vi "main.vi"() -> ()   [LabVIEW 2021]
uses:
  Controls/App Data Cluster.ctl
  Controls/UI Reference Cluster.ctl
  Controls/Database Variables Cluster.ctl
  <vilib>/drjdpowell/SQLite Library/SQL Connection/Connection.lvclass
  <vilib>/drjdpowell/SQLite Library/SQL Connection/Open (string).vi
  <extravilib>/ChannelInstances/Event Messenger-c(str,var)/Instantiate.vi
  <extravilib>/ChannelInstances/Event Messenger-c(str,var)/))Channel.vi
  <vilib>/drjdpowell/SQLite Library/SQL Connection/Execute SQL (1D DBL results).vi
  <vilib>/drjdpowell/SQLite Library/SQL Connection/Execute SQL (No results).vi
  <vilib>/Instr/_visa.llb/VISA Configure Serial Port (Instr).vi
  <extravilib>/ChannelInstances/Event Messenger-c(str,var).lvlib
  <vilib>/drjdpowell/SQLite Library/SQLite.lvlib
  <vilib>/JDP Science/JDP Science Common Utilities/JDP Utility.lvlib
panel:
  out "EndTime":string
  out "Result Set":dbl[](array[numeric])
  out "MDBUnit Test Result":cluster{"Message":string, "Passed?":bool}
  in  "Python script path":path=path "C:/Isaac/Projects/Mechanical Engineering Projects/LabVIEW Databases Project/LabVIEW-Databases/Python/mdb_helper.py"
  in  "Python install path":path=path "C:/Users/RIG/AppData/Local/Programs/Python/Python39-32/python.exe"
  out "SQLite Write Test Result":cluster{"Message":string, "Passed?":bool}
  in  "SQLite DB Path":string="C:\\Isaac\\Projects\\Mechanical Engineering Projects\\LabVIEW Databases Project\\SensorsDB.db"
  out "Serial Read Unit test results":cluster{"message":string, "Passed?":bool}[](array[cluster])
  out "App Data - Database Loop":T1
  out "error out":errorcluster
  in  "Save to MongoDB?":bool
  in  "Confirm details":bool
  in  "Save to SQLite?":bool
  in  "Start":bool
  in  "Stop":bool
  in  "Config run":bool
  in  "Select VISA resource name":refnum<visa-resource-name>
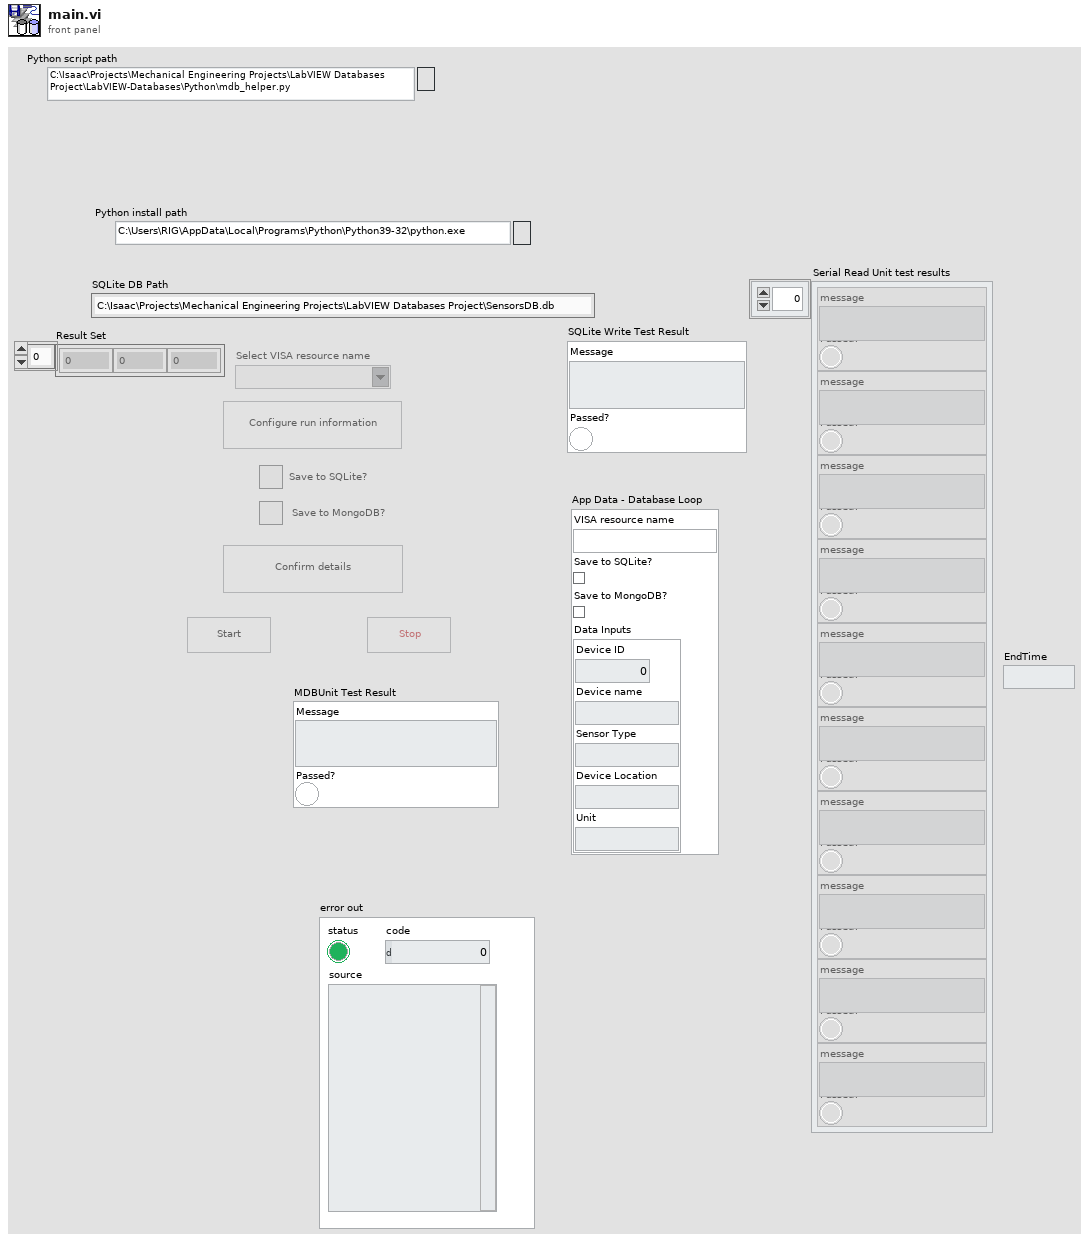
[diagram p1: front panel]
types:
  T1 = typedef "App Data Cluster.ctl" = cluster{"VISA resource name":refnum<visa-resource-name>, "Save to SQLite?":bool, "Save to MongoDB?":bool, "Data Inputs":cluster{"Device ID":dbl, "Device name":string, "Sensor Type":string, "Device Location":string, "Unit":string}}
  T2 = typedef "Database Variables Cluster.ctl" = cluster{"SQLite Connection":refnum<class "Connection.lvclass">, "Python Session":refnum<k35>, "Duplicate SQLite?":bool, "Duplicate MongoDB?":bool, "Start Time":string}
  T3 = typedef "UI Reference Cluster.ctl" = cluster{"Select VISA resource name":refnum<vi>, "Config run":refnum<vi>, "Save to SQLite":refnum<vi>, "Save to MongoDB":refnum<vi>, "Confirm details":refnum<vi>, "Start":refnum<vi>, "Stop":refnum<vi>}
  T4 = typedef "Event Messenger-c(str,var).lvlib/))Channel.ctl" = refnum<queue>
  T5 = cluster{"Device ID":dbl, "Device name":string, "Sensor Type":string, "Device Location":string, "Unit":string}
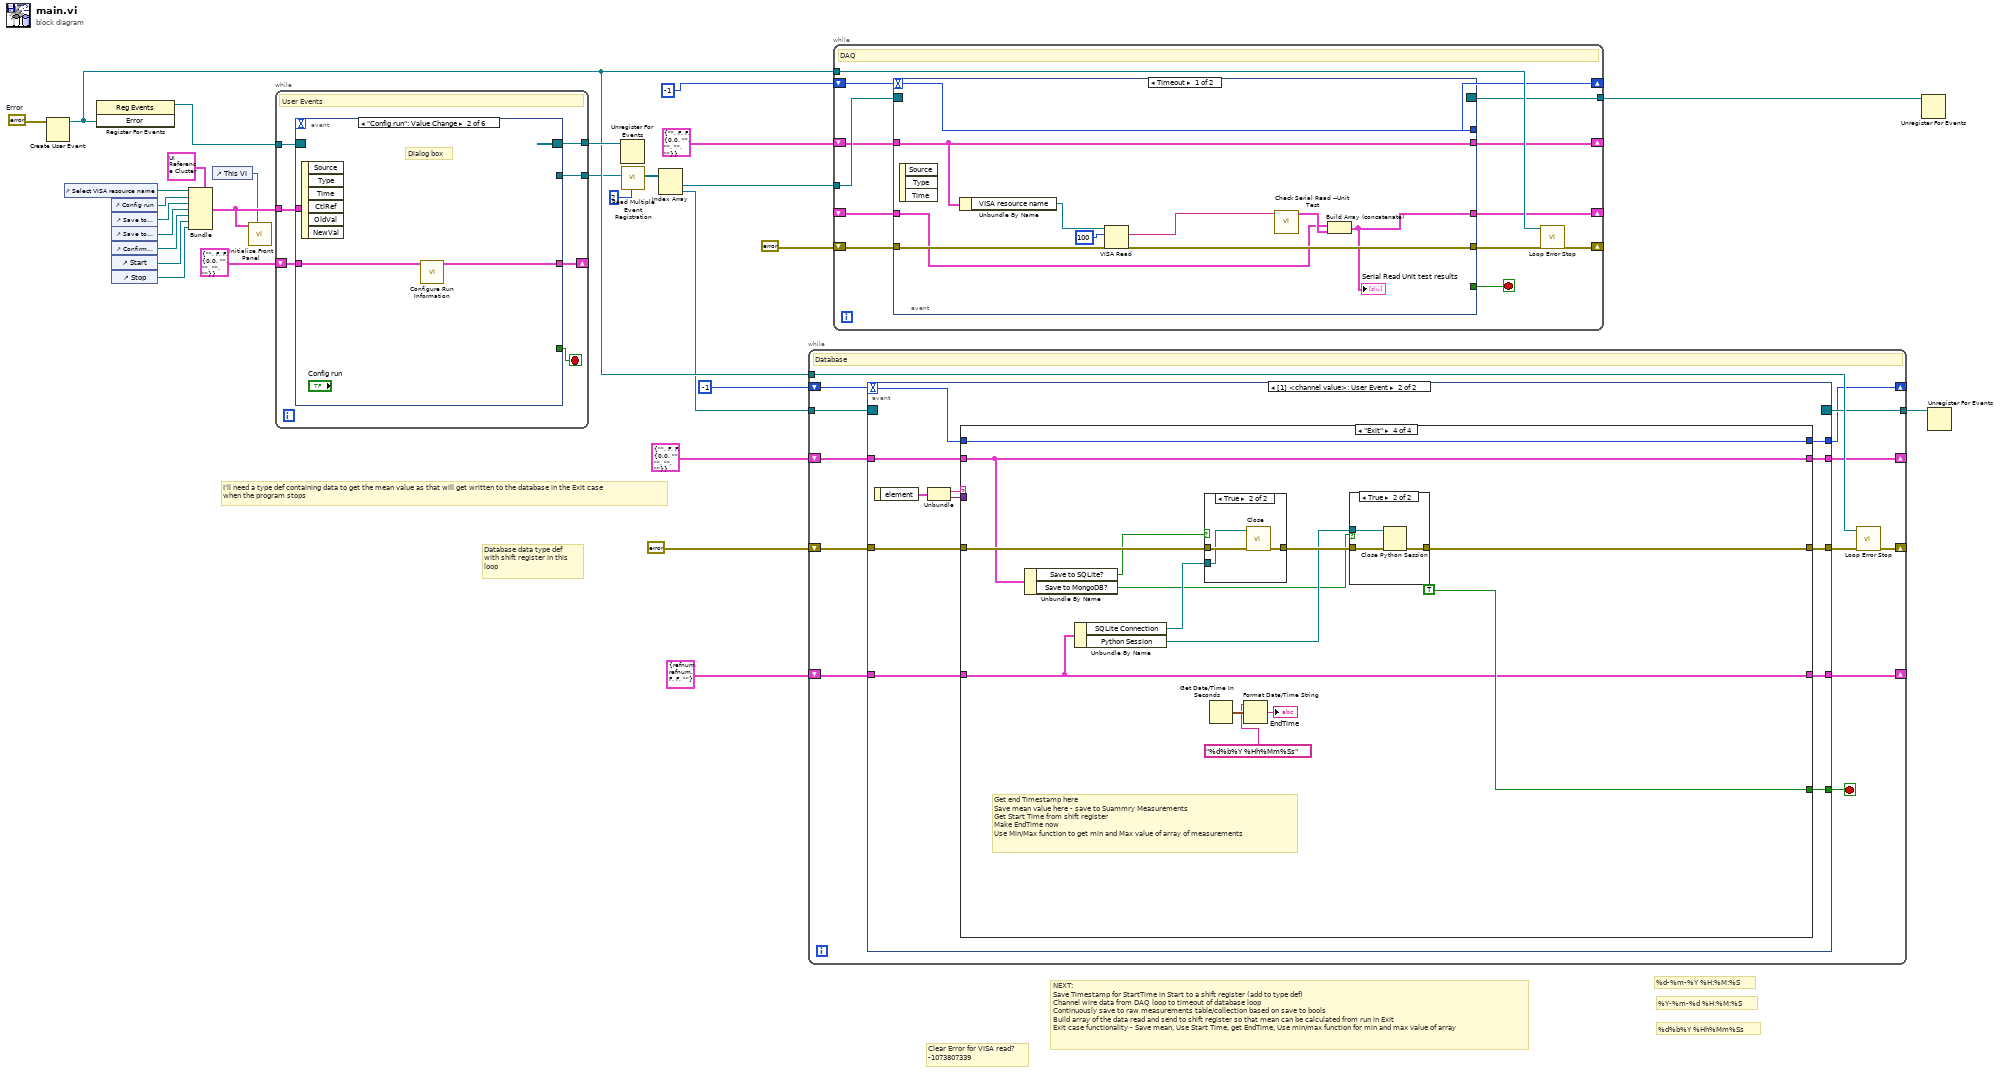
[diagram p0: block diagram]
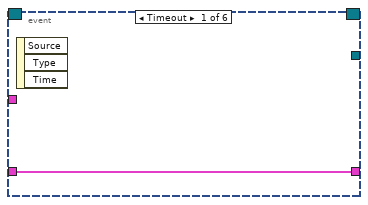
[diagram p2: hidden frame]
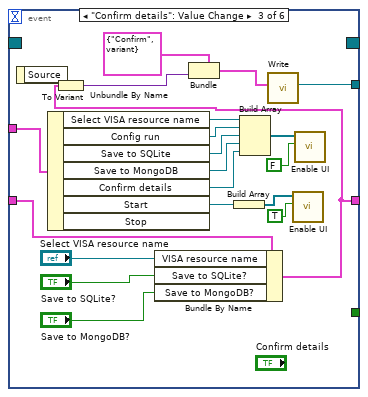
[diagram p3: hidden frame]
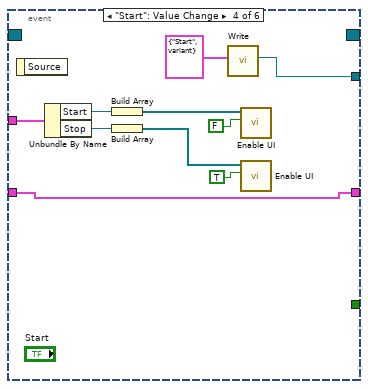
[diagram p4: hidden frame]
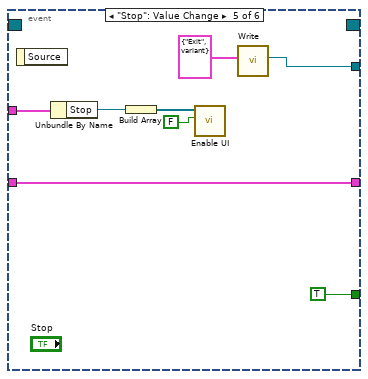
[diagram p5: hidden frame]
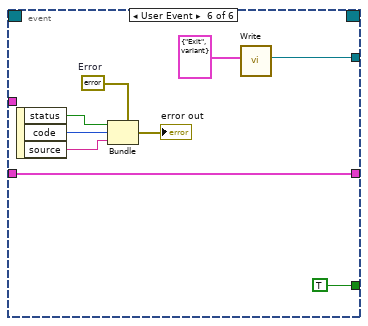
[diagram p6: hidden frame]
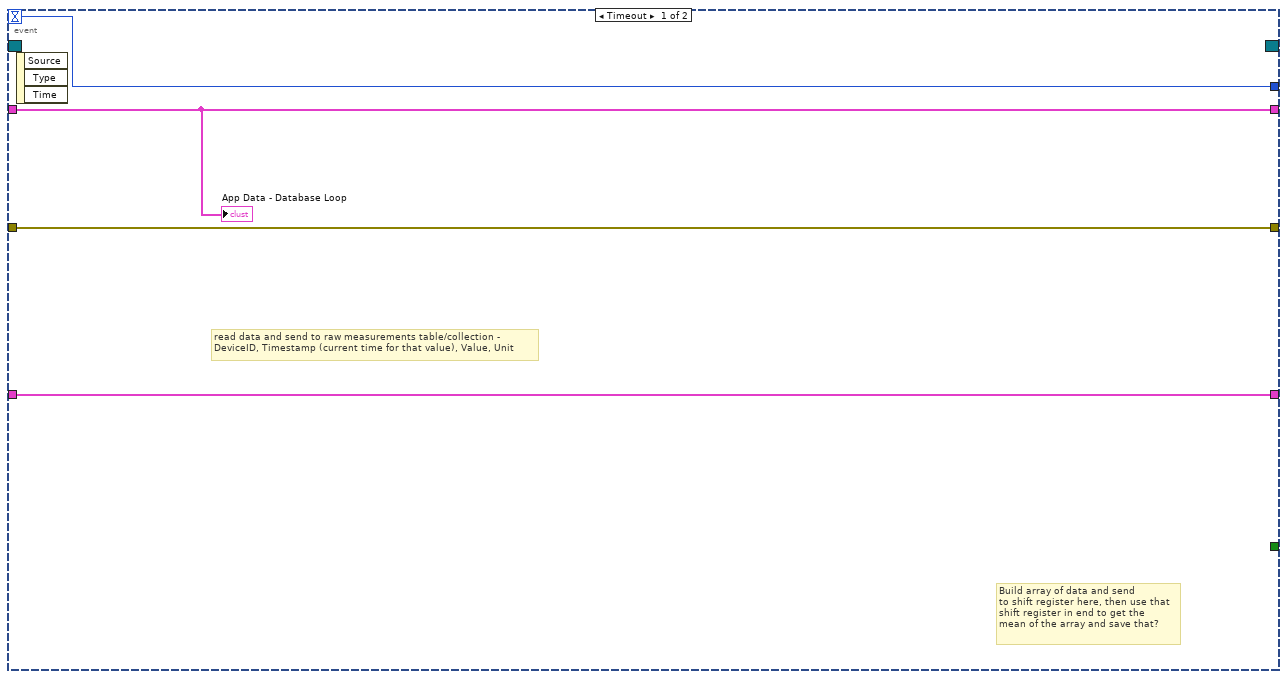
[diagram p7: hidden frame]
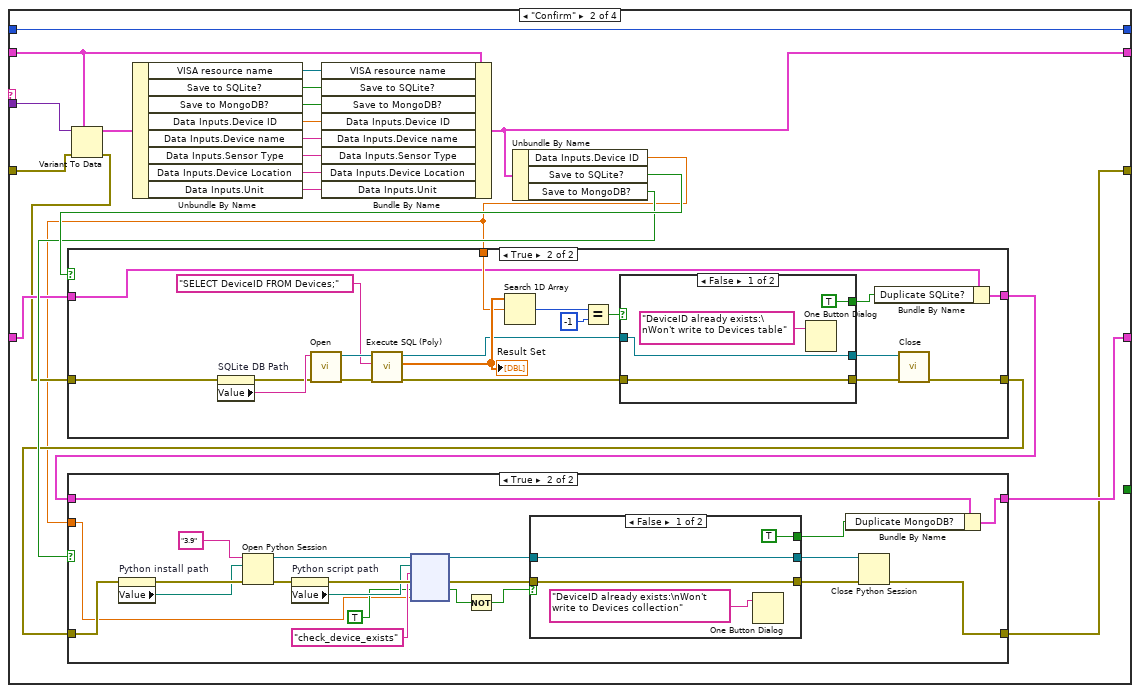
[diagram p9: hidden frame]
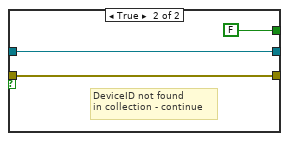
[diagram p11: hidden frame]
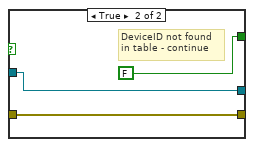
[diagram p13: hidden frame]
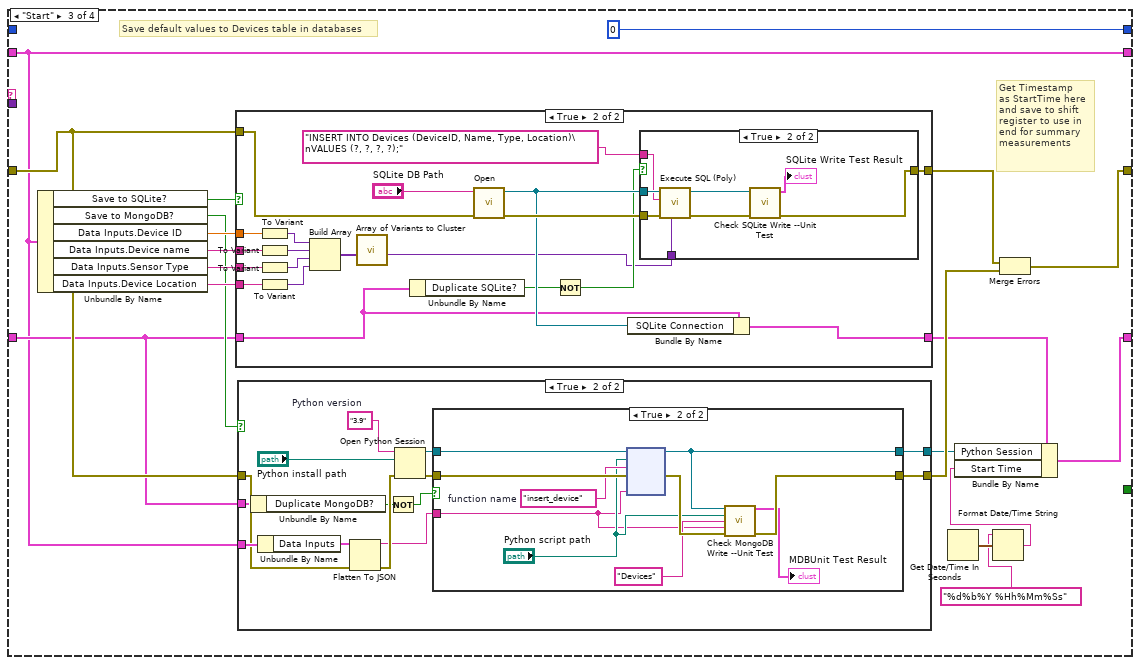
[diagram p14: hidden frame]
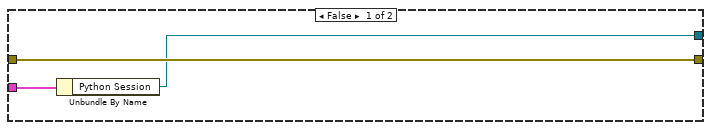
[diagram p15: hidden frame]
diagram:
  w22 = errorcluster {"status"=FALSE, "code"=0, "source"=""}  # Error
  # "%d-%m-%Y %H:%M:%S"
  # "%d%b%Y %Hh%Mm%Ss"
  # "%Y-%m-%d %H:%M:%S"
  # "Clear Error for VISA read?\n-1073807339"
  # "NEXT:\nSave Timestamp for StartTime in Start to a shift register (add to type def)\nChannel wire data from DAQ loop to timeout of database loop\nContinuously save to raw measurements table/collection based on save to bools\nBuild array of the data read and send to shift register so that mean can be calculated from run in Exit\nExit case functionality - Save mean, Use Start Time, get EndTime, Use min/max function for min and max value of array"
  # "Database data type def\nwith shift register in this \nloop"
  # "I'll need a type def containing data to get the mean value as that will get written to the database in the Exit case\nwhen the program stops"
  n1 = Create User Event(user event datatype=w22) -> (user event=w19:refnum<user-event>)  [unwired: 1 in, 1 out]
  n2 = control-ref of="Select VISA resource name"() -> (w29:refnum<vi>)
  n3 = register-events(w19) -> (reference out=w21:refnum<event-registration>)  [unwired: 2 in, 1 out]
  n4 = control-ref of="Config run"() -> (w28:refnum<vi>)
  n5 = control-ref of="Save to SQLite?"() -> (w27:refnum<vi>)
  n6 = control-ref of="Save to MongoDB?"() -> (w26:refnum<vi>)
  n7 = control-ref of="Confirm details"() -> (w25:refnum<vi>)
  n8 = control-ref of="Start"() -> (w24:refnum<vi>)
  n9 = control-ref of="Stop"() -> (w23:refnum<vi>)
  n10 = Bundle(cluster=T3 {"Select VISA resource name"=refnum, "Config run"=refnum, "Save to SQLite"=refnum, "Save to MongoDB"=refnum, "Confirm details"=refnum, "Start"=refnum, "Stop"=refnum} ("Output cluster"), "Select VISA resource name"=w29, "Config run"=w28, "Save to SQLite"=w27, "Save to MongoDB"=w26, "Confirm details"=w25, "Start"=w24, "Stop"=w23) -> (w15:T3)
  n11 = control-ref of="This VI"() -> (w14:refnum<vi>)
  n12 = call "Initialise Front Panel.vi"("This VI"=w14, "UI Ref"=w15) -> ()  [unwired: 9 in, 1 out]
  n13 = while {
    tunnel: w15 -> [w36]
    tunnel: w21 -> [w35]
    tunnel: [w34] -> w20
    tunnel: [w32] -> w13
    shift-right: [w31] -> _
    shift-left: T1 {"VISA resource name"="", "Save to SQLite?"=FALSE, "Save to MongoDB?"=FALSE, "Data Inputs"={"Device ID"=0.0, "Device name"="", "Sensor Type"="", "Device Location"="", "Unit"=""}} ("App Data") -> [w30]
    stop <- w33 stop-if-true
    # "User Events"
    n14 = event shown="[1] \"Config run\": Value Change" {
      selector: w35 -> [_ _ _ _ _ _]
      dyn-events: [_ _ _ _ _ _] -> w34
      timeout: _ -> [_ _ _ _ _ _]
      tunnel: w36 -> [_ _ w59 w69 w75 _]
      tunnel: [_ _ _ _ TRUE TRUE] -> w33
      tunnel: [_ _ w48 w61 w71 w79] -> w32
      tunnel: [w37 w38 w43 w60 w70 w78] -> w31
      tunnel: w30 -> [w37 w39 w47 w60 w70 w78]
      event Timeout {
        n15 = event-data() -> ()  [unwired: 1 in, 3 out]
      }
      event "Config run": Value Change {
        # "Dialog box"
        n16 = event-data() -> ()  [unwired: 1 in, 6 out]
        n17 = call "Configure Run Information.vi"("App Data In"=w39) -> ("App Data Out"=w38:T1)  [unwired: 9 in, 1 out]
      }
      event "Confirm details": Value Change {
        n18 = event-data() -> ()  [unwired: 1 in, 1 out]
        n19 = Unbundle By Name(w59) -> ("Select VISA resource name"=w58:refnum<vi>, "Config run"=w57:refnum<vi>, "Save to SQLite"=w56:refnum<vi>, "Save to MongoDB"=w55:refnum<vi>, "Confirm details"=w54:refnum<vi>, "Start"=w51:refnum<vi>)  [unwired: 1 out]
        n20 = Bundle By Name(cluster=w47, "VISA resource name"="Select VISA resource name", "Save to SQLite?"="Save to SQLite?", "Save to MongoDB?"="Save to MongoDB?") -> (w43:T1)
        n21 = To Variant(anything=w43) -> (Variant=w41:variant)
        n22 = Bundle(cluster=cluster{string, "Data":variant} {"Confirm", "Data"=variant}, "Data"=w41) -> (w40:cluster{string, "Data":variant})  [unwired: 1 in]
        n23 = Build Array(w51) -> (w50:refnum<vi>[])
        n24 = Build Array(w58, w57, w56, w55, w54) -> (w53:refnum<vi>[])
        n25 = call <extravilib>:"Write.vi"("element"=w40) -> ("channel"=w48:T4)  [unwired: 9 in, 1 out]
        n26 = call "Enable UI.vi"("Enable?"=TRUE, "output cluster"=w50) -> ()  [unwired: 9 in, 1 out]
        n27 = call "Enable UI.vi"("Enable?"=FALSE, "output cluster"=w53) -> ()  [unwired: 9 in, 1 out]
      }
      event "Start": Value Change {
        n28 = event-data() -> ()  [unwired: 1 in, 1 out]
        n29 = Unbundle By Name(w69) -> ("Start"=w68:refnum<vi>, "Stop"=w67:refnum<vi>)
        n30 = Build Array(w68) -> (w66:refnum<vi>[])
        n31 = Build Array(w67) -> (w65:refnum<vi>[])
        n32 = call <extravilib>:"Write.vi"("element"=cluster{string, "Data":variant} {"Start", "Data"=variant}) -> ("channel"=w61:T4)  [unwired: 9 in, 1 out]
        n33 = call "Enable UI.vi"("Enable?"=FALSE, "output cluster"=w66) -> ()  [unwired: 9 in, 1 out]
        n34 = call "Enable UI.vi"("Enable?"=TRUE, "output cluster"=w65) -> ()  [unwired: 9 in, 1 out]
      }
      event "Stop": Value Change {
        n35 = event-data() -> ()  [unwired: 1 in, 1 out]
        n36 = Unbundle By Name(w75) -> ("Stop"=w74:refnum<vi>)
        n37 = Build Array(w74) -> (w77:refnum<vi>[])
        n38 = call "Enable UI.vi"("Enable?"=FALSE, "output cluster"=w77) -> ()  [unwired: 9 in, 1 out]
        n39 = call <extravilib>:"Write.vi"("element"=cluster{string, "Data":variant} {"Exit", "Data"=variant}) -> ("channel"=w71:T4)  [unwired: 9 in, 1 out]
      }
      event User Event {
        w83 = errorcluster {"status"=FALSE, "code"=0, "source"=""}  # Error
        n40 = event-data() -> ("status"=w86:bool, "code"=w85:i32, "source"=w84:string)  [unwired: 1 in]
        n41 = Bundle(cluster=w83, "status"=w86, "code"=w85, "source"=w84) -> (→"error out":errorcluster)
        n42 = call <extravilib>:"Write.vi"("element"=cluster{string, "Data":variant} {"Exit", "Data"=variant}) -> ("channel"=w79:T4)  [unwired: 9 in, 1 out]
      }
    }
  }
  n43 = Unregister For Events(event registration refnum=w20) -> ()  [unwired: 1 in, 1 out]
  n44 = call <extravilib>:"Read Multiple Event Registration.vi"("number of event structures"=u16 2, "channel"=w13) -> ("event registration refnums"=w11:refnum<event-registration>[])  [unwired: 9 in]
  n45 = Index Array(array=w11) -> (element #1=w10:refnum<event-registration>, element #2=w9:refnum<event-registration>)  [unwired: 2 in]
  n46 = while {
    tunnel: w19 -> [w99]
    tunnel: [w98] -> w17
    tunnel: w9 -> [w97]
    shift-right: [w95] -> _
    shift-left: -1 -> [w96]
    shift-right: [w93] -> _
    shift-left: T1 {"VISA resource name"="", "Save to SQLite?"=FALSE, "Save to MongoDB?"=FALSE, "Data Inputs"={"Device ID"=0.0, "Device name"="", "Sensor Type"="", "Device Location"="", "Unit"=""}} ("App Data") -> [w94]
    shift-right: [w91] -> _
    shift-left: errorcluster {"status"=FALSE, "code"=0, "source"=""} ("error constant") -> [w90]
    shift-right: [w87] -> _
    shift-left: T2 {"SQLite Connection"=refnum, "Python Session"=refnum, "Duplicate SQLite?"=FALSE, "Duplicate MongoDB?"=FALSE, "Start Time"=""} ("Database variables") -> [w88]
    stop <- w92 stop-if-true
    # "Database"
    n47 = event shown="[1] <channel value>: User Event" {
      selector: w97 -> [_ _]
      dyn-events: [_ _] -> w98
      timeout: w96 -> [w103 w113]
      tunnel: [w103 w112] -> w95
      tunnel: w94 -> [w102 w111]
      tunnel: [w102 w110] -> w93
      tunnel: [_ w109] -> w92
      tunnel: w90 -> [w101 w107]
      tunnel: [w101 w106] -> w89
      tunnel: w88 -> [w100 w105]
      tunnel: [w100 w104] -> w87
      event Timeout {
        # "read data and send to raw measurements table/collection - \nDeviceID, Timestamp (current time for that value), Value, Unit"
        # "Build array of data and send \nto shift register here, then use that\nshift register in end to get the \nmean of the array and save that?"
        n48 = event-data() -> ()  [unwired: 1 in, 3 out]
        "App Data - Database Loop" <- w102
      }
      event User Event {
        n49 = event-data() -> ("element"=w115:cluster{string, "Data":variant})  [unwired: 1 in]
        n50 = Unbundle(w115) -> (w114:string, "Data"=w108:variant)
        n51 = case shown="\"Exit\"" w114 {
          tunnel: [_ _ _ TRUE] -> w109
          tunnel: w113 -> [w119 w142 _ w292]
          tunnel: [w119 w142 0 w292] -> w112
          tunnel: w111 -> [w118 w140 w205 w285]
          tunnel: [w118 w129 w205 w285] -> w110
          tunnel: w108 -> [_ w141 _ _]
          tunnel: w107 -> [w117 w135 w212 w289]
          tunnel: [w117 w121 w209 w287] -> w106
          tunnel: w105 -> [w116 w126 w206 w291]
          tunnel: [w116 w122 w207 w291] -> w104
          frame Default {
          }
          frame "Confirm" {
            n52 = Variant To Data(error in=w135, type=w140, Variant=w141) -> (data=w139:T1, error out=w125:errorcluster)
            n53 = Unbundle By Name(w139) -> ("VISA resource name"=w138:refnum<visa-resource-name>, "Save to SQLite?"=w137:bool, "Save to MongoDB?"=w136:bool, "Data Inputs.Device ID"=w134:dbl, "Data Inputs.Device name"=w133:string, "Data Inputs.Sensor Type"=w132:string, "Data Inputs.Device Location"=w131:string, "Data Inputs.Unit"=w130:string)
            n54 = Bundle By Name(cluster=w140, "VISA resource name"=w138, "Save to SQLite?"=w137, "Save to MongoDB?"=w136, "Data Inputs.Device ID"=w134, "Data Inputs.Device name"=w133, "Data Inputs.Sensor Type"=w132, "Data Inputs.Device Location"=w131, "Data Inputs.Unit"=w130) -> (w129:T1)
            n55 = Unbundle By Name(w129) -> ("Data Inputs.Device ID"=w120:dbl, "Save to SQLite?"=w128:bool, "Save to MongoDB?"=w127:bool)
            n56 = case shown="True" w128 {
              tunnel: w125 -> [w173 w192]
              tunnel: w120 -> [_ w179]
              tunnel: [w173 w178] -> w124
              tunnel: w126 -> [w174 w177]
              tunnel: [w174 w176] -> w123
              frame False {
              }
              frame True {
                n57 = property on="SQLite DB Path" class="Str"(error in=w192) -> (error out=w190:errorcluster, "Value"=w191:string)  [unwired: 1 in, 1 out]
                n58 = call-poly <vilib>:"Open.vi"("error in (no error)"=w190, "db file"=w191) -> ("error out"=w193:errorcluster, "SQLite Connection"=w189:refnum<class "Connection.lvclass">)  [unwired: 8 in]
                n59 = call-poly <vilib>:"Execute SQL (Poly).vi"("error in (no error)"=w193, "SQL"="SELECT DeviceID FROM Devices;", "SQLite Connection in"=w189) -> ("error out"=w185:errorcluster, "Result Set"=w187:dbl[], "SQLite Connection"=w183:refnum<class "Connection.lvclass">)  [unwired: 5 in, 1 out]
                "Result Set" <- w187
                n60 = Search 1D Array(1D array=w187, element=w179) -> (index of element=w182:i32)  [unwired: 1 in]
                n61 = Equal?(x=w182, y=-1) -> (x = y?=w180:bool)
                n62 = case shown="False" w180 {
                  tunnel: [w196 w199] -> w186
                  tunnel: w185 -> [w196 w199]
                  tunnel: [w197 w200] -> w184
                  tunnel: w183 -> [w197 w200]
                  tunnel: [TRUE FALSE] -> w175
                  frame False {
                    n63 = One Button Dialog(message="DeviceID already exists:\nWon't write to Devices table" ("error source (\" \")")) -> ()  [unwired: 1 in, 1 out]
                  }
                  frame True {
                    # "DeviceID not found\nin table - continue"
                  }
                }
                n64 = Bundle By Name(cluster=w177, "Duplicate SQLite?"=w175) -> (w176:T2)
                n65 = call-dynamic "Close.vi"("error in (no error)"=w186, "SQLite Connection in"=w184) -> ("error out"=w178:errorcluster)  [unwired: 9 in]
              }
            }
            n66 = case shown="True" w127 {
              tunnel: w124 -> [w143 w165]
              tunnel: w123 -> [w144 w150]
              tunnel: [w144 w149] -> w122
              tunnel: [w143 w160] -> w121
              tunnel: w120 -> [_ w147]
              frame False {
              }
              frame True {
                n67 = property on="Python install path" class="Path"(error in=w165) -> (error out=w164:errorcluster, "Value"=w163:path)  [unwired: 1 in, 1 out]
                n68 = Open Python Session(python version="3.9" ("Python version"), python path=w163, 3:w164) -> (session out=w161:refnum<k35>, error out=w159:errorcluster)
                n69 = property on="Python script path" class="Path"(error in=w159) -> (error out=w158:errorcluster, "Value"=w157:path)  [unwired: 1 in, 1 out]
                n70 = node(w161, w157, "check_device_exists" ("function name"), w158, TRUE, w147) -> (w153:refnum<k35>, w154:errorcluster, w146:bool)  [unwired: 1 in, 2 out]
                n71 = Not(x=w146) -> (.not. x?=w145:bool)
                n72 = case shown="False" w145 {
                  tunnel: w154 -> [w168 w172]
                  tunnel: w153 -> [w167 w171]
                  tunnel: [w168 w172] -> w152
                  tunnel: [w167 w171] -> w151
                  tunnel: [TRUE FALSE] -> w148
                  frame False {
                    n73 = One Button Dialog(message="DeviceID already exists:\nWon't write to Devices collection" ("error source (\" \")")) -> ()  [unwired: 1 in, 1 out]
                  }
                  frame True {
                    # "DeviceID not found\nin collection - continue"
                  }
                }
                n74 = Bundle By Name(cluster=w150, "Duplicate MongoDB?"=w148) -> (w149:T2)
                n75 = Close Python Session(session in=w151, error in=w152) -> (11:w160:errorcluster)
              }
            }
          }
          frame "Start" {
            # "Get Timestamp\nas StartTime here\nand save to shift\nregister to use in\nend for summary \nmeasurements"
            # "Save default values to Devices table in databases"
            n76 = Unbundle By Name(w205) -> ("Save to SQLite?"=w218:bool, "Save to MongoDB?"=w213:bool, "Data Inputs.Device ID"=w217:dbl, "Data Inputs.Device name"=w216:string, "Data Inputs.Sensor Type"=w215:string, "Data Inputs.Device Location"=w214:string)
            n77 = case shown="True" w218 {
              tunnel: w212 -> [w250 w268]
              tunnel: [w250 w257] -> w210
              tunnel: w217 -> [_ w267]
              tunnel: w216 -> [_ w266]
              tunnel: w215 -> [_ w265]
              tunnel: w214 -> [_ w264]
              tunnel: w206 -> [w249 w255]
              tunnel: [w249 w258] -> w204
              frame False {
              }
              frame True {
                n78 = To Variant(anything=w267) -> (Variant=w263:variant)
                n79 = To Variant(anything=w266) -> (Variant=w262:variant)
                n80 = To Variant(anything=w265) -> (Variant=w261:variant)
                n81 = To Variant(anything=w264) -> (Variant=w260:variant)
                n82 = Build Array(w263, w262, w261, w260) -> (w259:variant[])
                n83 = call <vilib>:"Array of Variants to Cluster.vi"("Array of Variants"=w259) -> ("Cluster of Variants"=w251:variant)  [unwired: 10 in]
                n84 = Unbundle By Name(w255) -> ("Duplicate SQLite?"=w254:bool)
                n85 = call-poly <vilib>:"Open.vi"("error in (no error)"=w268, "db file"="SQLite DB Path") -> ("error out"=w269:errorcluster, "SQLite Connection"=w256:refnum<class "Connection.lvclass">)  [unwired: 8 in]
                n86 = Not(x=w254) -> (.not. x?=w253:bool)
                n87 = Bundle By Name(cluster=w255, "SQLite Connection"=w256) -> (w258:T2)
                n88 = case shown="True" w253 {
                  tunnel: w256 -> [_ w279]
                  tunnel: w269 -> [w271 w278]
                  tunnel: "INSERT INTO Devices (DeviceID, Name, Type, Location)\nVALUES (?, ?, ?, ?);" ("SQL") -> [_ w273]
                  tunnel: [w271 w276] -> w257
                  tunnel: w251 -> [_ w272]
                  frame False {
                    # "DeviceID already exists in table\ndon't write to Devices table again"
                  }
                  frame True {
                    n89 = call-poly <vilib>:"Execute SQL (Poly).vi"("Parameter(s)"=w272, "error in (no error)"=w278, "SQL"=w273, "SQLite Connection in"=w279) -> ("error out"=w277:errorcluster, "SQLite Connection"=w275:refnum<class "Connection.lvclass">)  [unwired: 6 in]
                    n90 = call "Check SQLite Write --Unit Test.vi"("error in"=w277, "SQLite Connection"=w275) -> ("error out"=w276:errorcluster, "Test Result"=→"SQLite Write Test Result":cluster{"Message":string, "Passed?":bool})  [unwired: 8 in]
                  }
                }
              }
            }
            n91 = case shown="True" w213 {
              tunnel: w212 -> [w222 w230]
              tunnel: [w222 w228] -> w211
              tunnel: [w220 w227] -> w208
              tunnel: w206 -> [w221 w226]
              tunnel: w205 -> [_ w232]
              frame False {
                n92 = Unbundle By Name(w221) -> ("Python Session"=w220:refnum<k35>)
              }
              frame True {
                w236 = "3.9"  # Python version
                n93 = Unbundle By Name(w226) -> ("Duplicate MongoDB?"=w224:bool)
                n94 = Unbundle By Name(w232) -> ("Data Inputs"=w231:T5)
                n95 = Flatten To JSON(anything=w231, error in (no error)=w230) -> (JSON string=w223:string, 11:w229:errorcluster)  [unwired: 1 in]
                n96 = Not(x=w224) -> (.not. x?=w225:bool)
                n97 = Open Python Session(python version=w236, python path="Python install path", 3:w229) -> (session out=w233:refnum<k35>, error out=w234:errorcluster)
                n98 = case shown="True" w225 {
                  tunnel: w234 -> [w237 w248]
                  tunnel: w233 -> [w238 w247]
                  tunnel: [w237 w244] -> w228
                  tunnel: [w238 w243] -> w227
                  tunnel: w223 -> [_ w240]
                  frame False {
                  }
                  frame True {
                    w246 = "insert_device"  # function name
                    n99 = node(w247, "Python script path", w246, w248, w240) -> (w243:refnum<k35>, w245:errorcluster)  [unwired: 3 in, 2 out]
                    n100 = call "Check MongoDB Write --Unit Test.vi"("Python Session"=w243, "Python script path"="Python script path", "Collection name"="Devices", "Expected JSON string"=w240, "error in"=w245) -> ("Unit Test Result"=→"MDBUnit Test Result":cluster{"Message":string, "Passed?":bool}, "error out"=w244:errorcluster)  [unwired: 9 in]
                  }
                }
              }
            }
            n101 = Get Date/Time In Seconds() -> (seconds since 1Jan1904=w203:timestamp)
            n102 = Format Date/Time String(time format string (%c)="%d%b%Y %Hh%Mm%Ss", seconds (now)=w203) -> (date/time string=w202:string)  [unwired: 1 in]
            n103 = Bundle By Name(cluster=w204, "Python Session"=w208, "Start Time"=w202) -> (w207:T2)
            n104 = Merge Errors(w210, w211) -> (w209:errorcluster)
          }
          frame "Exit" {
            # "Get end Timestamp here\nSave mean value here - save to Suammry Measurements\nGet Start Time from shift register\nMake EndTime now\nUse Min/Max function to get min and Max value of array of measurements"
            n105 = Unbundle By Name(w285) -> ("Save to SQLite?"=w284:bool, "Save to MongoDB?"=w283:bool)
            n106 = Unbundle By Name(w291) -> ("SQLite Connection"=w290:refnum<class "Connection.lvclass">, "Python Session"=w286:refnum<k35>)
            n107 = case shown="True" w284 {
              tunnel: w290 -> [_ w299]
              tunnel: w289 -> [w298 w301]
              tunnel: [w298 w300] -> w288
              frame False {
              }
              frame True {
                n108 = call-dynamic "Close.vi"("error in (no error)"=w301, "SQLite Connection in"=w299) -> ("error out"=w300:errorcluster)  [unwired: 9 in]
              }
            }
            n109 = Get Date/Time In Seconds() -> (seconds since 1Jan1904=w282:timestamp)
            n110 = Format Date/Time String(time format string (%c)="%d%b%Y %Hh%Mm%Ss", seconds (now)=w282) -> (date/time string=→"EndTime":string)  [unwired: 1 in]
            n111 = case shown="True" w283 {
              tunnel: w288 -> [w294 w297]
              tunnel: [w294 w296] -> w287
              tunnel: w286 -> [_ w295]
              frame False {
              }
              frame True {
                n112 = Close Python Session(session in=w295, error in=w297) -> (11:w296:errorcluster)
              }
            }
          }
        }
      }
    }
    n113 = call "Loop Error Stop.vi"("error in"=w89, "user event"=w99) -> ("error out"=w91:errorcluster)  [unwired: 9 in]
  }
  n114 = while {
    tunnel: w19 -> [w314]
    tunnel: [w313] -> w18
    tunnel: w10 -> [w312]
    shift-right: [w310] -> _
    shift-left: -1 -> [w311]
    shift-right: [w307] -> _
    shift-left: T1 {"VISA resource name"="", "Save to SQLite?"=FALSE, "Save to MongoDB?"=FALSE, "Data Inputs"={"Device ID"=0.0, "Device name"="", "Sensor Type"="", "Device Location"="", "Unit"=""}} ("App Data") -> [w309]
    shift-right: [w306] -> _
    shift-left: errorcluster {"status"=FALSE, "code"=0, "source"=""} ("error constant") -> [w305]
    shift-right: [w303] -> _
    shift-left: _ -> [w302]
    stop <- w308 stop-if-true
    # "DAQ"
    n115 = event shown="[0] Timeout" {
      selector: w312 -> [_ _]
      dyn-events: [_ _] -> w313
      timeout: w311 -> [w324 w332]
      tunnel: [w324 w333] -> w310
      tunnel: w309 -> [w322 w330]
      tunnel: [_ w331] -> w308
      tunnel: [w322 w329] -> w307
      tunnel: w305 -> [w323 w327]
      tunnel: [w319 w326] -> w304
      tunnel: [w317 w325] -> w303
      tunnel: w302 -> [w315 w325]
      event Timeout {
        n116 = event-data() -> ()  [unwired: 1 in, 3 out]
        n117 = Unbundle By Name(w322) -> ("VISA resource name"=w321:refnum<visa-resource-name>)
        n118 = VISA Read(VISA resource name=w321, byte count=u32 100, error in (no error)=w323) -> (read buffer=w318:string, error out=w319:errorcluster)  [unwired: 2 out]
        n119 = call "Check Serial Read --Unit Test.vi"("Read buffer In"=w318) -> ("Results out"=w316:cluster{"message":string, "Passed?":bool})  [unwired: 10 in]
        n120 = Build Array (concatenate)(w315, w316) -> (w317:cluster{"message":string, "Passed?":bool}[])
        "Serial Read Unit test results" <- w317
      }
      event User Event {
        n121 = event-data() -> ("element"=w335:cluster{string, "Data":variant})  [unwired: 1 in]
        n122 = Unbundle(w335) -> (w334:string, "Data"=w328:variant)
        n123 = case shown="\"Confirm\"" w334 {
          tunnel: [_ _ _ TRUE] -> w331
          tunnel: [w338 w353 0 w368] -> w333
          tunnel: w332 -> [w338 w353 _ w368]
          tunnel: w330 -> [w337 w350 w358 w365]
          tunnel: [w337 w352 w356 w365] -> w329
          tunnel: w328 -> [_ w351 _ _]
          tunnel: w327 -> [w336 w345 w355 w367]
          tunnel: [w336 w344 w354 w366] -> w326
          frame Default {
          }
          frame "Confirm" {
            n124 = Variant To Data(error in=w345, type=w350, Variant=w351) -> (data=w349:T1, error out=w344:errorcluster)
            n125 = Unbundle By Name(w349) -> ("VISA resource name"=w348:refnum<visa-resource-name>, "Save to SQLite?"=w347:bool, "Save to MongoDB?"=w346:bool, "Data Inputs.Device ID"=w343:dbl, "Data Inputs.Device name"=w342:string, "Data Inputs.Sensor Type"=w341:string, "Data Inputs.Device Location"=w340:string, "Data Inputs.Unit"=w339:string)
            n126 = Bundle By Name(cluster=w350, "VISA resource name"=w348, "Save to SQLite?"=w347, "Save to MongoDB?"=w346, "Data Inputs.Device ID"=w343, "Data Inputs.Device name"=w342, "Data Inputs.Sensor Type"=w341, "Data Inputs.Device Location"=w340, "Data Inputs.Unit"=w339) -> (w352:T1)
          }
          frame "Start" {
            n127 = Unbundle By Name(w358) -> ("VISA resource name"=w362:refnum<visa-resource-name>)
            n128 = call-poly "VISA Configure Serial Port"("VISA resource name"=w362, "baud rate (9600)"=u32 115200, "error in (no error)"=w355) -> ("VISA resource name out"=w361:refnum<visa-resource-name>, "error out"=w359:errorcluster)  [unwired: 11 in]
            n129 = VISA Flush I/O Buffer(VISA resource name=w361, error in (no error)=w359) -> (VISA resource name out=w357:refnum<visa-resource-name>, error out=w354:errorcluster)  [unwired: 1 in]
            n130 = Bundle By Name(cluster=w358, "VISA resource name"=w357) -> (w356:T1)
          }
          frame "Exit" {
            n131 = Unbundle By Name(w365) -> ("VISA resource name"=w364:refnum<visa-resource-name>)
            n132 = VISA Close(VISA resource name=w364, error in (no error)=w367) -> (error out=w366:errorcluster)
          }
        }
      }
    }
    n133 = call "Loop Error Stop.vi"("error in"=w304, "user event"=w314) -> ("error out"=w306:errorcluster)  [unwired: 9 in]
  }
  n134 = Unregister For Events(event registration refnum=w18) -> ()  [unwired: 1 in, 1 out]
  n135 = Unregister For Events(event registration refnum=w17) -> ()  [unwired: 1 in, 1 out]
